vi "Split block segments from line.vi"(2 "Input line string":string) -> (16 "Text segments":string[](array[string]))   [LabVIEW 2020]
doc: "Split line with spaces or equal signs into text segments."
panel:
  # "Split line with spaces or equal signs into text segments."
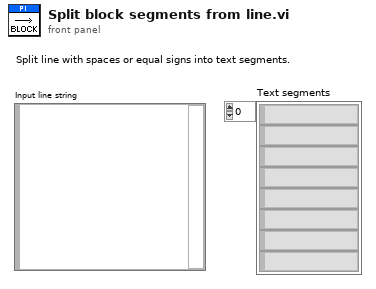
[diagram p1: front panel]
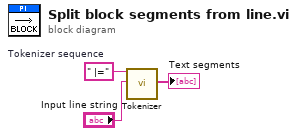
[diagram p0: block diagram]
diagram:
  w1 = " |="  # Tokenizer sequence
  n1 = call "Tokenizer.vi"("Tokenizer sequence"=w1, "Input string"="Input line string") -> ("Text segments"=→"Text segments":string[])  [unwired: 17 in]
